vi "Measure.vi"(6 "DevId":i32, 8 "error in":errorcluster caption="entrée d'erreur (pas d'erreur)", 9 "Scan":bool, 10 "IndicePoint":i32, 11 "Experiment.lvclass In":refnum<class "Experiment.lvclass">) -> (0 "error out":errorcluster caption="sortie d'erreur", 1 "ArrDevDat":T1[](array[typedef]), 2 "Données":dbl[](array[numeric]), 3 "Experiment.lvclass Out":refnum<class "Experiment.lvclass">, 4 "SaveArrVarPar":bool[](array[boolean]))   [LabVIEW 2019, in "Experiment.lvclass"]
uses:
  Experiment.lvclass
  ArrDevData.ctl
  Experiment.lvclass/Experiment.ctl
  DevicesClass/BaseDevice/BaseDevice.lvclass/BaseDevice.ctl
  DevicesClass/BaseDevice/GetSaveArrVarPar.vi
  DevicesClass/BaseDevice/BaseDevice.lvclass
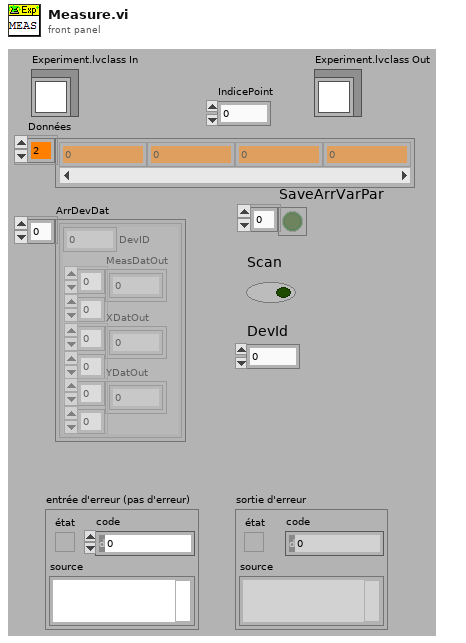
[diagram p1: front panel]
types:
  T1 = typedef "ArrDevData.ctl" = cluster{"MeasDatOut":dbl[][], "XDatOut":dbl[][], "YDatOut":dbl[][], "DevID":i32}
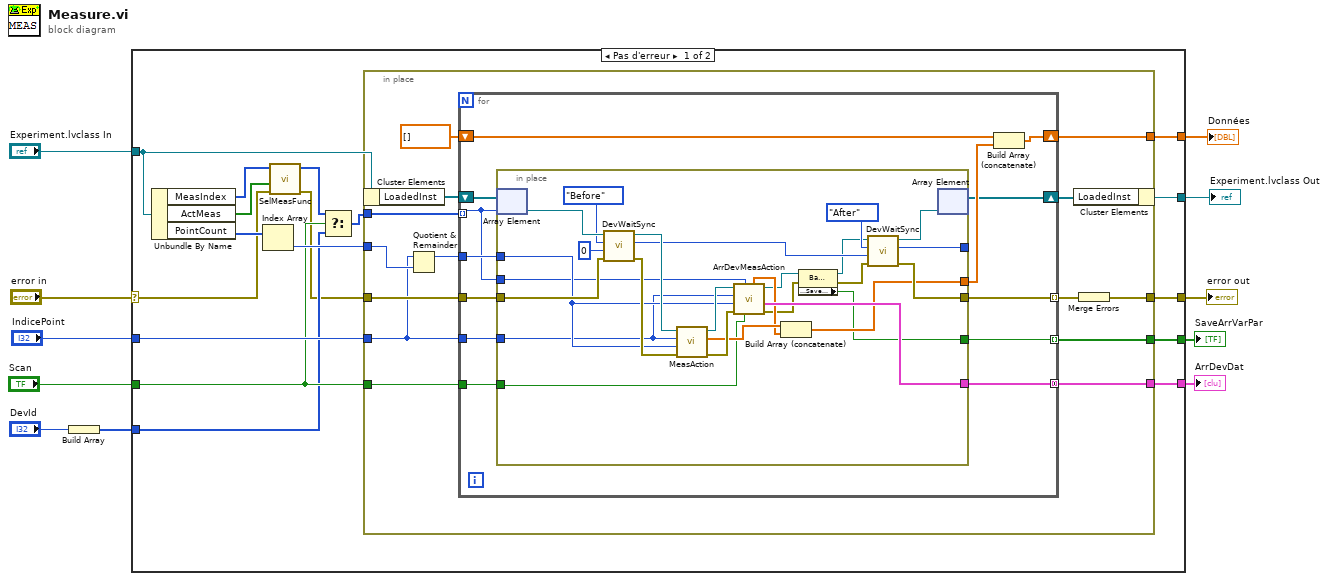
[diagram p0: block diagram]
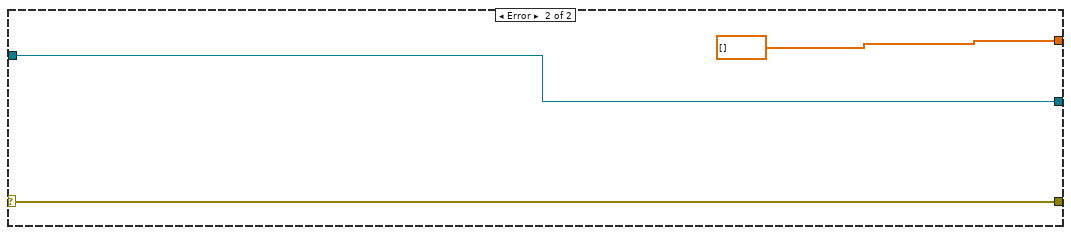
[diagram p2: hidden frame]
diagram:
  n1 = Build Array("DevId") -> (w1:i32[])
  n2 = case shown="Pas d'erreur" "error in" {
    selector: "error in" -> [w13 w84]
    tunnel: [w26 w84] -> w10
    tunnel: [w28 dbl[] [] ("Outputs")] -> w9
    tunnel: "IndicePoint" -> [w27 _]
    tunnel: "Experiment.lvclass In" -> [w25 w82]
    tunnel: [w24 w82] -> w6
    tunnel: [w21 _] -> w5
    tunnel: [w20 _] -> w4
    tunnel: "Scan" -> [w19 _]
    tunnel: w1 -> [w18 _]
    frame No Error {
      n3 = Unbundle By Name(w25) -> ("MeasIndex"=w15:i32[], "ActMeas"=w14:bool[], "PointCount"=w23:i32[])
      n4 = Index Array(array=w23) -> (element=w22:i32)  [unwired: 1 in]
      n5 = call "SelMeasFunc.vi"("ErrorIn(No Error)"=w13, "Active MeasPar"=w14, "MeasIndexIn"=w15) -> ("sortie d'erreur"=w12:errorcluster, "MeasIndexOut"=w16:i32[])  [unwired: 6 in, 1 out]
      n6 = Select(t=w16, s=w19, f=w18) -> (s? t:f=w17:i32[])
      n7 = in-place {
        in-place-border: w12 -> [w42]
        in-place-border: [w41] -> w28
        in-place-border: w27 -> [w33]
        in-place-border: [w39] -> w26
        in-place-border: w17 -> [w37]
        in-place-border: w22 -> [w34]
        in-place-border: [w31] -> w21
        in-place-border: [w30] -> w20
        in-place-border: w19 -> [w29]
        n8 = in-place-cluster #1(w25) -> ("LoadedInst"=w36:refnum<class "BaseDevice.lvclass">[])
        n9 = Quotient & Remainder(x=w33, y=w34) -> (x-y*floor(x/y)=w32:i32)  [unwired: 1 out]
        n10 = for {
          tunnel: w42 -> [w52]
          tunnel: w33 -> [w53]
          shift-right: [w55] -> w41
          shift-left: dbl[] [] -> [w54]
          tunnel: [w51] -> w38 mode=indexing
          tunnel: w37 -> [w46] mode=indexing
          shift-right: [w48] -> w35
          shift-left: w36 -> [w49]
          tunnel: w32 -> [w47]
          tunnel: [w45] -> w31 mode=concatenating
          tunnel: [w44] -> w30 mode=indexing
          tunnel: w29 -> [w43]
          n11 = in-place {
            in-place-border: w53 -> [w67]
            in-place-border: w52 -> [w76]
            in-place-border: [w80] -> w51
            in-place-border: [w64] -> w50
            in-place-border: w47 -> [w68]
            in-place-border: [w71] -> _
            in-place-border: w46 -> [w65]
            in-place-border: [w66] -> w45
            in-place-border: [w60] -> w44
            in-place-border: w43 -> [w56]
            n12 = in-place-array #2(w49, w46) -> (w78:refnum<class "BaseDevice.lvclass">)
            n13 = call "DevWaitSync.vi"("error in (no error)"=w76, "Time in"=u32 0, "Type"=enum16{"After", "Before"}."Before", "BaseDevice en entrée"=w78) -> ("error out"=w75:errorcluster, "Time"=w73:u32, "BaseDevice en sortie"=w77:refnum<class "BaseDevice.lvclass">)  [unwired: 5 in]
            n14 = call-dynamic "MeasAction.vi"("error in (no error)"=w75, "CurvePointIndex"=w68, "AllPointIndex"=w67, "Device In"=w77) -> ("error out"=w70:errorcluster, "MeasDatOut"=w63:dbl[], "Device Out"=w69:refnum<class "BaseDevice.lvclass">)  [unwired: 5 in]
            n15 = call-dynamic "ArrDevMeasAction.vi"("Scan"=w56, "DevId"=w65, "error in (no error)"=w70, "CurvePointIndex"=w68, "AllPointIndex"=w67, "Device In"=w69) -> ("error out"=w58:errorcluster, "ArrDevDat"=w66:T1[], "Device Out"=w59:refnum<class "BaseDevice.lvclass">, "MeasOut"=w62:dbl[])  [unwired: 1 in, 1 out]
            n16 = Build Array (concatenate)(w63, w62) -> (w64:dbl[])
            n17 = property class="BaseDevice.lvclass"(reference=w59, error in=w58) -> (reference out=w61:refnum<class "BaseDevice.lvclass">, error out=w57:errorcluster, "Accessor:SaveArrVarPar"=w60:bool)
            n18 = call "DevWaitSync.vi"("error in (no error)"=w57, "Time in"=w73, "Type"=enum16{"After", "Before"}."After", "BaseDevice en entrée"=w61) -> ("error out"=w80:errorcluster, "Time"=w71:u32, "BaseDevice en sortie"=w81:refnum<class "BaseDevice.lvclass">)  [unwired: 5 in]
            n19 = in-place-array #2(w81) -> (w48:refnum<class "BaseDevice.lvclass">[])  [unwired: 1 out]
          }
          n20 = Build Array (concatenate)(w54, w50) -> (w55:dbl[])
        }
        n21 = in-place-cluster #1("LoadedInst"=w35) -> (w24:refnum<class "Experiment.lvclass">)
        n22 = Merge Errors(w38) -> (w39:errorcluster)
      }
    }
    frame Error {
    }
  }
  "error out" <- w10
  "Données" <- w9
  "Experiment.lvclass Out" <- w6
  "ArrDevDat" <- w5
  "SaveArrVarPar" <- w4
